vi "循环发送CAN1.vi"(8 "错误输入":errorcluster caption="错误输出") -> (0 "错误输出":errorcluster)   [LabVIEW 2020]
uses:
  Libraries/ZLG_CAN/CAN_CYCLE.vi
  Libraries/ZLG_CAN/ZLG_CAN.lvlib
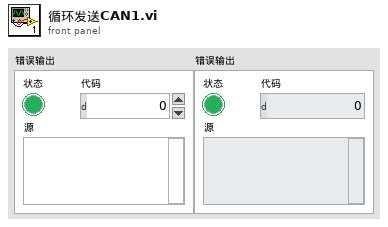
[diagram p1: front panel]
types:
  T1 = cluster{"ID":u32, "帧类型":enum8{"标准帧", "扩展帧"}, "帧格式":enum16{"数据帧", "远程帧"}, "帧数据":string, "周期(ms)":u32}[]
  T2 = enum32{"Invalid", "Standard", "Closed", "Hidden", "Minimized", "Maximized"}
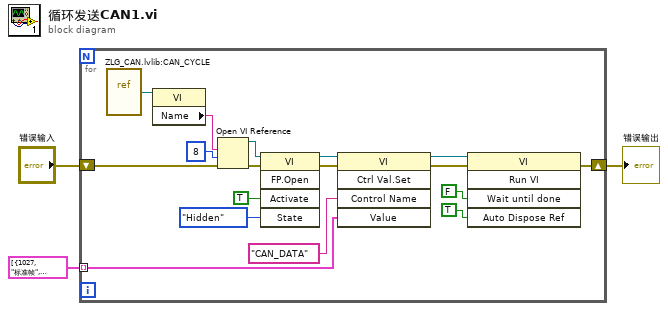
[diagram p0: block diagram]
diagram:
  n1 = for {
    tunnel: T1 [{"ID"=1027, "帧类型"=enum."标准帧", "帧格式"=enum."数据帧", "帧数据"="00 20 00 00 00 00 00 00", "周期(ms)"=10}] ("CAN_CYCLE") -> [w14] mode=indexing
    shift-right: [w6] -> w2
    shift-left: "错误输入" -> [w17]
    n2 = vi-ref "ZLG_CAN.lvlib:CAN_CYCLE.vi"() -> (w20:refnum<vi>)
    n3 = property class="VI"(reference=w20) -> ("Name"=w19:string)  [unwired: 1 in, 2 out]
    n4 = Open VI Reference(vi path=w19, options=8 ("选项"), error in (no error)=w17) -> (vi reference=w16:refnum<vi>, error out=w12:errorcluster)  [unwired: 3 in]
    n5 = invoke class="VI" method="FP.Open"(reference=w16, error in=w12, "Activate"=TRUE ("激活？"), "State"=T2."Hidden" ("状态")) -> (reference out=w13:refnum<vi>, error out=w11:errorcluster)  [unwired: 1 in, 3 out]
    n6 = invoke class="VI" method="Ctrl Val.Set"(reference=w13, error in=w11, "Control Name"="CAN_DATA" ("控件名"), "Value"=w14) -> (reference out=w8:refnum<vi>, error out=w7:errorcluster)  [unwired: 1 in, 3 out]
    n7 = invoke class="VI" method="Run VI"(reference=w8, error in=w7, "Wait until done"=FALSE ("结束前等待"), "Auto Dispose Ref"=TRUE ("自动销毁引用")) -> (error out=w6:errorcluster)  [unwired: 1 in, 4 out]
  }
  "错误输出" <- w2
